vi "KI6221.vi"() -> ()   [LabVIEW 2025] (continued)
                                tunnel: w2439 -> [w2628]
                                tunnel: w2438 -> [w2627]
                                tunnel: w2437 -> [w2626]
                                tunnel: w2436 -> [w2614]
                                tunnel: w2435 -> [w2622]
                                tunnel: [w2620] -> w2433
                                tunnel: w2432 -> [w2619]
                                tunnel: w2430 -> [w2618]
                                tunnel: [w2617] -> w2429
                                tunnel: w2428 -> [w2616]
                                tunnel: w2427 -> [w2615]
                                tunnel: [w2608] -> w2425
                                tunnel: w2421 -> [w2607]
                                tunnel: [w2607] -> w2420
                                tunnel: w2419 -> [w2606]
                                tunnel: [w2605] -> w2410
                                tunnel: [w2604] -> w2418
                                tunnel: [w2603] -> w2417
                                tunnel: [w2598] -> w2416
                                tunnel: w2415 -> [w2598]
                                tunnel: w2406 -> [w2597]
                                frame #0 {
                                # "set STEP source"
                                n1197 = Increment(x=w2465) -> (x+1=w2466:i32)
                                n1198 = case shown="0, Default" w2472 {
                                tunnel: w2471 -> [w2477 _]
                                tunnel: w2470 -> [w2476 _]
                                tunnel: w2469 -> [w2480 w2503]
                                tunnel: w2468 -> [w2479 _]
                                tunnel: [w2478 w2503] -> w2467
                                tunnel: w2464 -> [w2475 _]
                                tunnel: w2466 -> [w2474 _]
                                frame 0, Default {
                                n1199 = case shown="True" w2475 {
                                tunnel: w2480 -> [w2488 w2493]
                                tunnel: w2479 -> [w2487 w2495]
                                tunnel: [w2486 w2494] -> w2478
                                tunnel: w2477 -> [w2484 _]
                                tunnel: w2476 -> [w2483 _]
                                tunnel: w2474 -> [_ w2496]
                                frame False {
                                # "Set Source"
                                n1200 = Number To Exponential String(number=w2488) -> (E-format string=w2491:string)  [unwired: 3 in]
                                n1201 = Initialize Array(w2491, 1 ("dimension size")) -> (w2489:string[])
                                n1202 = call "VisaVarReplace.vi"("Replace Array"=w2489, "Search Array"=string[] ["<LEVEL>"], "GPIB Array"=w2484) -> ("GPIB Array OUT"=w2482:string[])
                                n1203 = call "VISAreadWrite.vi"("GPIB INDEX Array"=i32[] [2], "GPIB ARRAY"=w2482, "VISA REFERENCE"=w2483) -> ("error out 15"=→"error out 23":errorcluster)  [unwired: 1 in, 1 out]
                                n1204 = Add(x=w2488, y=w2487) -> (x+y=w2486:dbl)
                                }
                                frame True {
                                n1205 = Number To Decimal String(number=w2496) -> (decimal integer string=w2498:string)  [unwired: 1 in]
                                n1206 = Number To Engineering String(4:w2493) -> (0:w2497:string)  [unwired: 3 in]
                                n1207 = Concatenate Strings("Please set the external step source for sweep number " ("y"), w2498, ". The correct source setting should be " ("y"), w2497, "." ("string")) -> (w2499:string)
                                n1208 = call "STEP SETUP"("Message"=w2499) -> ()  [unwired: 9 in, 2 out]
                                n1209 = Add(x=w2493, y=w2495) -> (x+y=w2494:dbl)
                                }
                                }
                                }
                                frame 2 {
                                # "No source"
                                }
                                }
                                }
                                frame #1 {
                                # "WORK AUTO TEST or \nFORWARD current values"
                                n1210 = case shown="0, Default" w2522 {
                                tunnel: w2521 -> [w2537 _]
                                tunnel: w2520 -> [_ w2595]
                                tunnel: w2519 -> [_ w2596]
                                tunnel: w2518 -> [_ w2591]
                                tunnel: w2517 -> [w2536 _]
                                tunnel: w2516 -> [w2535 _]
                                tunnel: w2515 -> [w2534 _]
                                tunnel: [w2533 w2592] -> w2514
                                tunnel: [w2532 w2595] -> w2507
                                tunnel: [w2531 w2596] -> w2506
                                tunnel: [w2530 w2591] -> w2513
                                tunnel: w2512 -> [w2529 _]
                                tunnel: w2511 -> [w2528 _]
                                tunnel: w2510 -> [w2527 w2590]
                                tunnel: [w2526 w2590] -> w2509
                                tunnel: [w2525 TRUE ("CONTINUE")] -> w2508
                                tunnel: w2505 -> [w2524 _]
                                tunnel: w2504 -> [w2523 _]
                                frame 0, Default {
                                # "voltage"
                                n1211 = case shown="0, Default" w2537 {
                                tunnel: w2536 -> [w2559 w2588]
                                tunnel: w2535 -> [w2558 w2586]
                                tunnel: w2534 -> [w2557 w2580]
                                tunnel: [w2555 w2581] -> w2533
                                tunnel: [w2549 w2583] -> w2532
                                tunnel: [w2556 w2582] -> w2531
                                tunnel: [w2557 w2580] -> w2530
                                tunnel: w2529 -> [w2554 _]
                                tunnel: w2528 -> [w2553 _]
                                tunnel: w2527 -> [w2552 w2579]
                                tunnel: [w2548 w2579] -> w2526
                                tunnel: [w2547 TRUE ("CONTINUE")] -> w2525
                                tunnel: w2524 -> [w2546 _]
                                tunnel: w2523 -> [w2545 _]
                                frame 0, Default {
                                # "auto test"
                                n1212 = flat-sequence {
                                tunnel: w2553 -> [w2561]
                                tunnel: w2554 -> [w2562]
                                tunnel: w2557 -> [w2563]
                                tunnel: w2558 -> [w2564]
                                tunnel: [w2564] -> w2544
                                tunnel: [w2563] -> w2543
                                tunnel: [w2562] -> w2542
                                tunnel: [w2561] -> w2541
                                tunnel: w2559 -> [w2577]
                                tunnel: [w2574] -> w2556
                                tunnel: [w2573] -> w2555
                                tunnel: [w2572] -> w2539
                                tunnel: w2552 -> [w2569]
                                tunnel: [w2568] -> w2549
                                tunnel: [w2567] -> w2547
                                tunnel: w2546 -> [w2566]
                                tunnel: w2545 -> [w2565]
                                tunnel: w2544 -> [w2576]
                                tunnel: w2543 -> [w2575]
                                tunnel: w2542 -> [w2571]
                                tunnel: w2541 -> [w2570]
                                frame #0 {
                                n1213 = property on="auto test \nlabel" class="Str"("Visible"=TRUE) -> ()  [unwired: 2 in, 2 out]
                                }
                                frame #1 {
                                n1214 = call "autotest.vi"("6220 VISA"=w2571, "start v"=w2577, "stop v"=w2576, "numPTS"=w2575, "GPIB Array"=w2570, "AUTO ARRAY"=w2569, "INIT start I"=w2566, "INIT stop I"=w2565) -> ("start I"=w2568:dbl, "stop I"=w2574:dbl, "step I"=w2573:dbl, "CONTINUE"=w2567:bool, "error out 15"=w2572:errorcluster)  [unwired: 3 in]
                                }
                                }
                                n1215 = property on="auto test label" class="Str"(error in=w2539, "Visible"=FALSE) -> (error out=→"error out 29":errorcluster)  [unwired: 1 in, 1 out]
                                n1216 = Number To Engineering String(4:w2549) -> (0:w2550:string)  [unwired: 3 in]
                                n1217 = Replace Array Subset(array=w2552, new element=w2550, index=4) -> (w2548:string[])
                                }
                                frame 1 {
                                # "estimated res"
                                n1218 = property on="Resistance in Ohms" class="DigNum (strict)"() -> ("Value"=w2587:dbl)  [unwired: 2 in, 2 out]
                                n1219 = Decrement(x=w2580) -> (x-1=w2584:i32)
                                n1220 = Divide(x=w2588, y=w2587) -> (x/y=w2583:dbl)
                                n1221 = Divide(x=w2586, y=w2587) -> (x/y=w2582:dbl)
                                n1222 = Subtract(x=w2582, y=w2583) -> (x-y=w2585:dbl)
                                n1223 = Divide(x=w2585, y=w2584) -> (x/y=w2581:dbl)
                                }
                                }
                                }
                                frame 1 {
                                # "current setup"
                                n1224 = Decrement(x=w2591) -> (x-1=w2593:i32)
                                n1225 = Subtract(x=w2596, y=w2595) -> (x-y=w2594:dbl)
                                n1226 = Divide(x=w2594, y=w2593) -> (x/y=w2592:dbl)
                                }
                                }
                                }
                                frame #2 {
                                # "PING every 3 sec. for all data in buffer. When it is ready grab data, parse into data sheet, and select columns for GRAPHS"
                                # "SEND SCPI CONFIG"
                                # "CREATE VISA SCPI STRINGS"
                                # "DC delta\nsetting\n\nstepsize"
                                # "run sweep"
                                n1227 = Number To Exponential String(number=w2599) -> (E-format string=w2621:string)  [unwired: 3 in]
                                n1228 = Number To Exponential String(number=w2599) -> (E-format string=w2633:string)  [unwired: 3 in]
                                n1229 = local read "Setup String"() -> (w2602:string)
                                n1230 = call "DCONSweepFix.vi"("NUM PTS"=w2614, "STEP"=w2599, "STOP"=w2610, "START"=w2613) -> ("Source Array"=w2609:dbl[], "STOP 2"=w2611:dbl, "START 2"=w2612:dbl)
                                n1231 = Not(x=w2606) -> (.not. x?=w2605:bool)
                                n1232 = Number To Exponential String(number=w2611) -> (E-format string=w2634:string)  [unwired: 3 in]
                                n1233 = Number To Exponential String(number=w2612) -> (E-format string=w2635:string)  [unwired: 3 in]
                                n1234 = Insert Into Array(array=string[] [], new element=w2635) -> (w2645:string[])  [unwired: 1 in]
                                n1235 = Insert Into Array(array=w2645, new element=w2634) -> (w2644:string[])  [unwired: 1 in]
                                n1236 = Insert Into Array(array=w2644, new element=w2633) -> (w2643:string[])  [unwired: 1 in]
                                n1237 = Insert Into Array(array=w2643, new element=w2632) -> (w2639:string[])  [unwired: 1 in]
                                n1238 = Insert Into Array(array=w2639, new element=w2621) -> (w2642:string[])  [unwired: 1 in]
                                n1239 = Insert Into Array(array=w2642, new element=w2631) -> (w2641:string[])  [unwired: 1 in]
                                n1240 = Insert Into Array(array=w2641, new element=w2630) -> (w2640:string[])  [unwired: 1 in]
                                n1241 = Insert Into Array(array=w2640, new element=w2629) -> (w2636:string[])  [unwired: 1 in]
                                n1242 = Insert Into Array(array=w2636, new element=w2628) -> (w2638:string[])  [unwired: 1 in]
                                n1243 = Insert Into Array(array=w2638, new element=w2627) -> (w2637:string[])  [unwired: 1 in]
                                n1244 = Insert Into Array(array=w2637, new element=w2626) -> (w2600:string[])  [unwired: 1 in]
                                n1245 = Insert Into Array(array=w2600, new element=w2602) -> (w2601:string[])  [unwired: 1 in]
                                n1246 = call "VisaVarReplace.vi"("Replace Array"=w2601, "Search Array"=string[] ["<DCONSTART>", "<DCONSTOP>", "<DCONSTEP>", "<DCONDELAY>", "<DCONDELTA>", "<DCONCOMP>", "<DCONDAMPING>", "<DCONVOLTRANGE>", "<DCONNPLC>", "<DCONFILTERSTATE>", "<DCONFILTERCOUNT>", "<SETUPSTRING>"], "GPIB Array"=w2623) -> ("GPIB Array OUT"=w2603:string[])
                                n1247 = case shown="True" w2606 {
                                tunnel: i32[] [24] -> [_ w2653]
                                tunnel: w2603 -> [_ w2652]
                                tunnel: [errorcluster {"status"=FALSE, "code"=0, "source"=""} ("error out 15") w2651] -> w2625
                                tunnel: w2604 -> [_ w2650]
                                frame False {
                                }
                                frame True {
                                n1248 = call "VISAreadWrite.vi"("GPIB INDEX Array"=w2653, "GPIB ARRAY"=w2652, "VISA REFERENCE"=w2650) -> ("error out 15"=w2651:errorcluster)  [unwired: 1 in, 1 out]
                                }
                                }
                                n1249 = case shown="No Error" w2625 {
                                tunnel: [w2672 TRUE ("ABORT DIFF COND")] -> w2624
                                tunnel: w2604 -> [w2671 _]
                                tunnel: w2623 -> [w2670 _]
                                tunnel: w2614 -> [w2669 _]
                                tunnel: w2622 -> [w2668 _]
                                tunnel: w2599 -> [w2667 _]
                                tunnel: [w2666 w2849] -> w2620
                                tunnel: w2619 -> [w2665 w2849]
                                tunnel: w2618 -> [w2664 _]
                                tunnel: [w2663 w2848] -> w2617
                                tunnel: w2616 -> [w2662 w2848]
                                tunnel: w2615 -> [w2661 _]
                                tunnel: w2609 -> [w2660 _]
                                tunnel: [w2659 errorcluster {"status"=FALSE, "code"=0, "source"=""} ("error out")] -> w2608
                                tunnel: w2605 -> [w2658 _]
                                tunnel: w2597 -> [w2656 _]
                                frame No Error {
                                n1250 = Multiply(x=w2656, y=1000.0) -> (x*y=w2655:dbl)
                                n1251 = Wait (ms)(milliseconds to wait=w2655) -> (millisecond timer value=w2654:u32)
                                n1252 = while {
                                tunnel: ["ABORT DIFF COND"] -> w2672
                                tunnel: w2671 -> [w2689]
                                tunnel: w2670 -> [w2688]
                                tunnel: w2669 -> [w2687]
                                tunnel: w2668 -> [w2685]
                                tunnel: w2667 -> [w2684]
                                tunnel: [w2683] -> w2666
                                tunnel: w2665 -> [w2682]
                                tunnel: w2664 -> [w2681]
                                tunnel: [w2680] -> w2663
                                tunnel: w2662 -> [w2679]
                                tunnel: w2661 -> [w2678]
                                tunnel: w2660 -> [w2677]
                                tunnel: [w2676] -> w2659
                                tunnel: w2658 -> [w2673]
                                tunnel: w2654 -> [_]
                                stop <- w2690 stop-if-true
                                n1253 = Or(x=w2673, y="ABORT DIFF COND") -> (x .or. y?=w2674:bool)
                                n1254 = case shown="False" w2674 {
                                selector: w2674 -> [_ w2846]
                                tunnel: w2689 -> [w2707 _]
                                tunnel: w2688 -> [w2706 _]
                                tunnel: w2687 -> [w2705 _]
                                tunnel: [w2702 w2846] -> w2686
                                tunnel: w2685 -> [w2700 _]
                                tunnel: w2684 -> [w2699 _]
                                tunnel: [w2698 w2845] -> w2683
                                tunnel: w2682 -> [w2697 w2845]
                                tunnel: w2681 -> [w2696 _]
                                tunnel: [w2695 w2844] -> w2680
                                tunnel: w2679 -> [w2694 w2844]
                                tunnel: w2678 -> [w2693 _]
                                tunnel: w2677 -> [w2692 _]
                                tunnel: [w2691 errorcluster {"status"=FALSE, "code"=0, "source"=""} ("error out")] -> w2676
                                frame False {
                                n1255 = case shown="True" w2704 {
                                tunnel: w2703 -> [w2716 _]
                                tunnel: [w2715 TRUE] -> w2702
                                tunnel: w2701 -> [_ w2766]
                                tunnel: w2700 -> [_ w2763]
                                tunnel: w2699 -> [_ w2762]
                                tunnel: [w2714 w2749] -> w2698
                                tunnel: w2697 -> [w2714 w2761]
                                tunnel: w2696 -> [_ w2737]
                                tunnel: [w2713 w2734] -> w2695
                                tunnel: w2694 -> [w2713 w2731]
                                tunnel: w2693 -> [_ w2729]
                                tunnel: w2692 -> [_ w2728]
                                tunnel: [w2712 w2724] -> w2691
                                tunnel: [w2711 w2720] -> _
                                tunnel: [w2711 w2719] -> _
                                tunnel: [w2711 w2718] -> _
                                frame False {
                                w2711 = dbl[] []
                                # "NO DATA"
                                n1256 = call "DATA QUERY ERROR"("Enable"=w2716) -> ("error out"=w2712:errorcluster, "Abort test now"=w2715:bool)  [unwired: 9 in]
                                }
                                frame True {
                                # "data"
                                n1257 = property on="Trace offset (% Pk-Pk):" class="DigNum (strict)"() -> ("Value"=w2742:dbl)  [unwired: 2 in, 2 out]
                                n1258 = Multiply(x=6, y=w2737) -> (x*y=w2759:i32)
                                n1259 = Divide(x=w2742, y=100.0) -> (x/y=w2740:dbl)
                                n1260 = Spreadsheet String To Array(delimiter (Tab)=",", format string="%e", spreadsheet string=w2766, array type (2D Dbl)=dbl[] []) -> (array=w2764:dbl[])
                                n1261 = property on="Horizontal Axis:" class="Ring (strict)"() -> ("Value"=w2754:u16)  [unwired: 2 in, 2 out]
                                n1262 = property on="Vertical Axis:" class="Ring (strict)"() -> ("Value"=w2756:u16)  [unwired: 2 in, 2 out]
                                n1263 = Add(x=w2756, y=u16 2) -> (x+y=w2748:u16)
                                n1264 = property on="Differential Conductance Graph" class="XYGraph (strict)"() -> ("Value"=w2757:cluster{"Y":dbl[], "Y":dbl[]}[])  [unwired: 2 in, 2 out]
                                n1265 = Unbundle(w2731) -> (w2733:dbl[], w2732:dbl[], w2730:dbl[])
                                n1266 = while {
                                tunnel: w2764 -> [w2783]
                                shift-right: [w2789] -> w2717
                                shift-left: string[][] [] -> [w2784]
                                tunnel: w2763 -> [w2779]
                                tunnel: w2762 -> [w2777]
                                tunnel: w2728 -> [w2771]
                                i -> [w2773]
                                stop <- w2801 stop-if-true
                                w2780 = "," ("delimiter (Tab)")
                                n1267 = Array Size(array=w2784) -> (size(s)=w2787:i32[])
                                n1268 = Index Array(array=w2787, index=0) -> (element=w2785:i32)
                                n1269 = Multiply(x=5, y=w2785) -> (x*y=w2804:i32)
                                n1270 = Index Array(array=w2783, index=w2804) -> (element=w2778:dbl)
                                n1271 = Divide(x=w2778, y=w2777) -> (x/y=w2776:dbl)
                                n1272 = Increment(x=w2804) -> (x+1=w2802:i32)
                                n1273 = Index Array(array=w2783, index=w2802) -> ()  [unwired: 1 out]
                                n1274 = Increment(x=w2802) -> (x+1=w2803:i32)
                                n1275 = Reciprocal(x=w2776) -> (1/x=w2790:dbl)
                                n1276 = Index Array(array=w2783, index=w2803) -> ()  [unwired: 1 out]
                                n1277 = Index Array(array=w2771, index=w2773) -> (element=w2772:dbl)
                                n1278 = Increment(x=w2803) -> (x+1=w2800:i32)
                                n1279 = Array Size(array=w2783) -> (size(s)=w2788:i32)
                                n1280 = Index Array(array=w2783, index=w2800) -> (element=w2774:dbl)
                                n1281 = Increment(x=w2800) -> (x+1=w2782:i32)
                                n1282 = Number To Engineering String(4:w2772) -> (0:w2794:string)  [unwired: 3 in]
                                n1283 = Number To Engineering String(4:w2776) -> (0:w2792:string)  [unwired: 3 in]
                                n1284 = Number To Engineering String(4:w2790) -> (0:w2791:string)  [unwired: 3 in]
                                n1285 = Number To Engineering String(4:w2778) -> (0:w2793:string)  [unwired: 3 in]
                                n1286 = Number To Engineering String(4:w2779) -> (0:w2775:string)  [unwired: 3 in]
                                n1287 = Number To Engineering String(4:w2774) -> (0:w2795:string)  [unwired: 3 in]
                                n1288 = Index Array(array=w2783, index=w2782) -> ()  [unwired: 1 out]
                                n1289 = Increment(x=w2782) -> (x+1=w2781:i32)
                                n1290 = Concatenate Strings(w2795, w2780, w2794, w2780, w2793, w2780, w2792, w2780, w2791, w2780, w2775) -> (w2796:string)
                                n1291 = Greater Or Equal?(x=w2781, y=w2788) -> (x >= y?=w2801:bool)
                                n1292 = Spreadsheet String To Array(delimiter (Tab)=w2780, format string="%s", spreadsheet string=w2796, array type (2D Dbl)=string[] []) -> (array=w2797:string[])
                                n1293 = Insert Into Array(array=w2784, index (row)=w2773, new element=w2797) -> (w2789:string[][])  [unwired: 1 in]
                                }
                                n1294 = Insert Into Array(array=w2761, index (col)=w2759, new element=w2717) -> (w2749:string[][])  [unwired: 1 in]
                                n1295 = Index Array(array=w2749, index (col)=w2748) -> (element=w2747:string[])  [unwired: 1 in]
                                n1296 = Fract/Exp String To Number(string=w2747) -> (number=w2746:dbl[])  [unwired: 3 in, 1 out]
                                n1297 = Array Max & Min(array=w2746) -> (max value=w2745:dbl, min value=w2744:dbl)  [unwired: 2 out]
                                n1298 = Subtract(x=w2745, y=w2744) -> (x-y=w2743:dbl)
                                n1299 = property on="Differential Conductance Measurement Data" class="Tbl (strict)"("Value"=w2749) -> ()  [unwired: 2 in, 2 out]
                                n1300 = Index Array(array=w2717, index (col)=w2754) -> (element=w2753:string[])  [unwired: 1 in]
                                n1301 = Index Array(array=w2717, index (col)=5 ("disabled index (col)")) -> (element=w2735:string[])  [unwired: 1 in]
                                n1302 = Fract/Exp String To Number(string=w2735) -> (number=w2726:dbl[])  [unwired: 3 in, 1 out]
                                n1303 = Index Array(array=w2717, index (col)=w2748) -> (element=w2752:string[])  [unwired: 1 in]
                                n1304 = Fract/Exp String To Number(string=w2752) -> (number=w2725:dbl[])  [unwired: 3 in, 1 out]
                                n1305 = Multiply(x=w2743, y=w2740) -> (x*y=w2739:dbl)
                                n1306 = Fract/Exp String To Number(string=w2753) -> (number=w2727:dbl[])  [unwired: 3 in, 1 out]
                                n1307 = Insert Into Array(array=w2733, new element=w2727) -> (w2719:dbl[])  [unwired: 1 in]
                                n1308 = Insert Into Array(array=w2732, new element=w2725) -> (w2718:dbl[])  [unwired: 1 in]
                                n1309 = Insert Into Array(array=w2730, new element=w2726) -> (w2720:dbl[])  [unwired: 1 in]
                                n1310 = Multiply(x=w2737, y=w2739) -> (x*y=w2738:dbl)
                                n1311 = Add(x=w2738, y=w2725) -> (x+y=w2750:dbl[])
                                n1312 = To Variant(anything=w2719) -> (Variant=w2722:variant)
                                n1313 = To Variant(anything=w2718) -> (Variant=w2721:variant)
                                n1314 = Bundle(w2727, w2750) -> (w2751:cluster{dbl[], dbl[]})  [unwired: 1 in]
                                n1315 = Insert Into Array(array=w2757, new element=w2751) -> (w2758:cluster{"Y":dbl[], "Y":dbl[]}[])  [unwired: 1 in]
                                n1316 = property on="Differential Conductance Graph" class="XYGraph (strict)"("Value"=w2758) -> ()  [unwired: 2 in, 2 out]
                                n1317 = To Variant(anything=w2720) -> (Variant=w2723:variant)
                                n1318 = Bundle(w2719, w2718, w2720) -> (w2734:cluster{dbl[], dbl[], dbl[]})  [unwired: 1 in]
                                n1319 = call "Stub 3d Graph-4.vi"("Variant"=w2721, "Variant 2"=w2722, "Variant 3"=w2723, "Differential Conductance Surface Plot"=w2729) -> ("error out"=w2724:errorcluster)
                                }
                                }
                                n1320 = flat-sequence {
                                tunnel: w2706 -> [w2808]
                                tunnel: w2707 -> [w2809]
                                tunnel: [w2809] -> w2710
                                tunnel: [w2808] -> w2709
                                tunnel: [w2807] -> w2708
                                tunnel: w2705 -> [w2807]
                                tunnel: [w2822] -> w2701
                                tunnel: w2710 -> [w2821]
                                tunnel: w2709 -> [w2812]
                                tunnel: w2708 -> [w2811]
                                tunnel: [w2814] -> w2704
                                tunnel: [w2813] -> w2703
                                frame #0 {
                                n1321 = Wait (ms)(milliseconds to wait=u32 3000) -> ()  [unwired: 1 out]
                                }
                                frame #1 {
                                n1322 = call "VISAreadWrite.vi"("GPIB INDEX Array"=i32[] [4], "GPIB ARRAY"=w2812, "VISA REFERENCE"=w2821) -> ("error out 15"=w2819:errorcluster, "Read Buffer Array"=w2817:string[])  [unwired: 1 in]
                                n1323 = Index Array(array=w2817, index=1) -> (element=w2816:string)
                                n1324 = Number To Decimal String(number=w2811) -> (decimal integer string=w2810:string)  [unwired: 1 in]
                                n1325 = Decimal String To Number(string=w2816) -> (number=w2815:i32)  [unwired: 2 in, 1 out]
                                n1326 = Less Or Equal?(x=w2811, y=w2815) -> (x <= y?=w2813:bool)
                                n1327 = case shown="True" w2813 {
                                tunnel: ["" w2837] -> w2822
                                tunnel: [FALSE w2836] -> w2814
                                tunnel: w2821 -> [_ w2832]
                                tunnel: w2819 -> [_ w2831]
                                tunnel: w2812 -> [_ w2830]
                                tunnel: w2810 -> [_ w2825]
                                frame False {
                                }
                                frame True {
                                n1328 = Insert Into Array(array=string[] [] ("Replace Array"), new element=w2825) -> (w2826:string[])  [unwired: 1 in]
                                n1329 = call "VisaVarReplace.vi"("Replace Array"=w2826, "Search Array"=string[] ["<DATACOUNT>"], "GPIB Array"=w2830) -> ("GPIB Array OUT"=w2829:string[])
                                n1330 = call "VISAreadWrite.vi"("error in (no error)"=w2831, "GPIB INDEX Array"=i32[] [23], "GPIB ARRAY"=w2829, "VISA REFERENCE"=w2832) -> ("error out 15"=w2834:errorcluster, "Read Buffer Array"=w2835:string[])
                                "error out 25" <- w2834
                                n1331 = Index Array(array=w2835, index=1) -> (element=w2837:string)
                                n1332 = Unbundle(w2834) -> ("source"=w2833:string)  [unwired: 2 out]
                                n1333 = Match Pattern(string=w2833, regular expression="-1073807339") -> (offset past match=w2841:i32)  [unwired: 1 in, 3 out]
                                n1334 = Equal?(x=w2841, y=-1) -> (x = y?=w2836:bool)
                                }
                                }
                                }
                                }
                                }
                                frame True {
                                }
                                }
                                n1335 = Compound Arithmetic op=OR(w2686, "ABORT DIFF COND") -> (w2690:bool)
                                }
                                }
                                frame Error {
                                }
                                }
                                }
                                }
                                n1336 = Decrement(x=w2463) -> (x-1=w2431:i32)
                                n1337 = Greater Or Equal?(x=w2430, y=w2431) -> (x >= y?=w2462:bool)
                                n1338 = Compound Arithmetic op=OR(w2412, w2462, w2410) -> (w2451:bool)
                                n1339 = Or(x=w2410, y=w2412) -> (x .or. y?=w2411:bool)
                                n1340 = Absolute Value(x=w2416) -> (abs(x)=w2408:dbl)
                                n1341 = Absolute Value(x=w2414) -> (abs(x)=w2407:dbl)
                                }
                                n1342 = property on="Main Tabs" class="TabCtl (strict)"(error in=w2236, "Page Selector Visible"=w2235) -> (error out=w2237:errorcluster)  [unwired: 1 in, 1 out]
                                n1343 = property on="Advanced Operation Tab" class="TabCtl (strict)"(error in=w2237, "Page Selector Visible"=w2235) -> (error out=w2279:errorcluster)  [unwired: 1 in, 1 out]
                                n1344 = while {
                                shift-right: [w2367] -> w2299
                                shift-left: string[] [] -> [w2368]
                                tunnel: string[] ["Voltage", "Current", "Delta Voltage", "Resistance", "Conductance", "Step Level"] -> [w2366]
                                tunnel: w2285 -> [w2362]
                                i -> [w2365]
                                stop <- w2363 stop-if-true
                                n1345 = Build Array (concatenate)(w2368, w2366) -> (w2367:string[])
                                n1346 = Increment(x=w2365) -> (x+1=w2364:i32)
                                n1347 = Equal?(x=w2364, y=w2362) -> (x = y?=w2363:bool)
                                }
                                n1348 = case shown="False" w2271 {
                                tunnel: w2279 -> [w2348 w2352]
                                tunnel: [w2348 w2351] -> w2257
                                tunnel: w2278 -> [_ w2350]
                                tunnel: w2277 -> [_ w2349]
                                frame False {
                                }
                                frame True {
                                n1349 = call "VISAreadWrite.vi"("error in (no error)"=w2352, "GPIB INDEX Array"=i32[] [3], "GPIB ARRAY"=w2349, "VISA REFERENCE"=w2350) -> ("error out 15"=w2351:errorcluster)  [unwired: 1 out]
                                }
                                }
                                n1350 = property on="Differential Conductance Measurement Data" class="Tbl (strict)"("Column Header Strings[]"=w2299) -> ()  [unwired: 2 in, 2 out]
                                n1351 = Equal To 0?(x=w2273) -> (x = 0?=w2288:bool)
                                n1352 = Greater?(x=w2285, y=1) -> (0:w2286:bool)
                                n1353 = And(x=w2288, y=w2286) -> (x .and. y?=w2289:bool)
                                n1354 = property on="DC TABS" class="TabCtl (strict)"() -> (error out=w2292:errorcluster, "Pages"=w2295:refnum<vi>[], "Value"=w2282:enum32{"2-D GRAPH", "3-D PLOT", "SHEET", "HELP"})  [unwired: 2 in, 1 out]
                                n1355 = Equal?(x=w2282, y=enum32{"2-D GRAPH", "3-D PLOT", "SHEET", "HELP"}."3-D PLOT") -> (x = y?=w2280:bool)
                                n1356 = case shown="False" w2289 {
                                tunnel: [2 ("y") 0 ("y")] -> w2287
                                tunnel: w2282 -> [w2355 w2360]
                                tunnel: [w2354 w2360] -> w2283
                                tunnel: w2280 -> [w2356 _]
                                frame False {
                                n1357 = case shown="True" w2356 {
                                tunnel: w2355 -> [w2358 _]
                                tunnel: [w2358 0 ("y")] -> w2354
                                frame False {
                                }
                                frame True {
                                }
                                }
                                }
                                frame True {
                                }
                                }
                                n1358 = call "VISAreadWrite.vi"("error in (no error)"=w2257, "GPIB INDEX Array"=i32[] [25], "GPIB ARRAY"=w2254, "VISA REFERENCE"=w2258) -> ("error out 15"=→"error out 32":errorcluster)  [unwired: 1 out]
                                n1359 = case shown="False" w2234 {
                                tunnel: w2244 -> [w2337 _]
                                frame False {
                                n1360 = Array Subset(array=w2337, index (col)=2 ("index"), length (col)=1 ("length")) -> (w2346:string[][])  [unwired: 2 in]
                                n1361 = Fract/Exp String To Number(string=w2346) -> (number=w2345:dbl[][])  [unwired: 3 in, 1 out]
                                n1362 = Array Max & Min(array=w2345) -> (max value=w2340:dbl, min value=w2344:dbl)  [unwired: 2 out]
                                n1363 = Greater?(x=w2340, y=1e+30) -> (0:w2338:bool)
                                n1364 = call "Volt range problem"("Enable"=w2338) -> ()  [unwired: 9 in, 2 out]
                                n1365 = Equal To 0?(x=w2340) -> (x = 0?=w2342:bool)
                                n1366 = Equal?(x=w2344, y=w2340) -> (x = y?=w2343:bool)
                                n1367 = And(x=w2343, y=w2342) -> (x .and. y?=w2341:bool)
                                n1368 = call "Volt range problem"("Enable"=w2341) -> ()  [unwired: 9 in, 2 out]
                                }
                                frame True {
                                }
                                }
                                n1369 = Index Array(array=w2295, index=1) -> (element=w2293:refnum<vi>)
                                n1370 = property class="Page"(reference=w2293, error in=w2292, "Page Enabled State"=w2287) -> (error out=w2291:errorcluster)  [unwired: 1 out]
                                n1371 = property on="DC TABS" class="TabCtl (strict)"(error in=w2291, "Value"=w2283) -> (error out=→"error out 30":errorcluster)  [unwired: 1 in, 1 out]
                              }
                            }
                          }
                        }
                      }
                      frame True {
                        # "DEMO MODE"
                        n1372 = property on="I want to control my\n test in terms of:" class="Ring (strict)"() -> ("Value"=w2862:u16)  [unwired: 2 in, 2 out]
                        n1373 = property on="Number of steps" class="DigNum (strict)"() -> ("Value"=w2861:i32)  [unwired: 2 in, 2 out]
                        n1374 = case shown="1" w2862 {
                          tunnel: [w2870 w2871] -> w2853
                          frame 0, Default {
                            n1375 = property on="Number of\n sweep points" class="DigNum (strict)"() -> ("Value"=w2870:i32)  [unwired: 2 in, 2 out]
                          }
                          frame 1 {
                            n1376 = property on="Number of\n sweep points" class="DigNum (strict)"() -> ("Value"=w2871:i32)  [unwired: 2 in, 2 out]
                          }
                        }
                        n1377 = Array Size(array=w2860) -> (size(s)=w2859:i32[])
                        n1378 = Index Array(array=w2859, index=0) -> (element=w2856:i32)
                        n1379 = Index Array(array=w2859, index=1) -> (element=w2855:i32)
                        n1380 = Initialize Array("", w2856, w2855) -> (w2863:string[][])
                        n1381 = while {
                          tunnel: w2869 -> [w2892]
                          tunnel: w2868 -> [w2877]
                          tunnel: w2860 -> [w2883]
                          tunnel: w2867 -> [w2891]
                          shift-right: [w2885] -> _
                          shift-left: w2863 -> [w2886]
                          tunnel: w2861 -> [w2873]
                          tunnel: w2854 -> [w2876]
                          tunnel: cluster{"Y":dbl[], "Y":dbl[]}[] [] ("XY Graph") -> [w2888]
                          tunnel: dbl[][] [] -> [w2884]
                          tunnel: w2853 -> [_]
                          tunnel: w2852 -> [w2874]
                          i -> [w2881]
                          stop <- w2889 stop-if-true
                          w2879 = 6 ("y")
                          n1382 = Multiply(x=w2881, y=w2879) -> (x*y=w2880:i32)
                          n1383 = Array Subset(array=w2883, index (col)=w2880, length (col)=w2879) -> (w2882:string[][])  [unwired: 2 in]
                          n1384 = Add(x=u16 2, y=w2892) -> (x+y=w2878:u16)
                          n1385 = Index Array(array=w2882, index (col)=w2877) -> (element=w2895:string[])  [unwired: 1 in]
                          n1386 = Index Array(array=w2882, index (col)=w2878) -> (element=w2894:string[])  [unwired: 1 in]
                          n1387 = Array Size(array=w2894) -> (size(s)=w2893:i32)
                          n1388 = case shown="True" w2891 {
                            tunnel: [u16 0 ("x") w2907] -> w2890
                            tunnel: [w2900 w2902] -> w2875
                            tunnel: string[] ["Voltage", "Current", "Delta Voltage", "Resistance", "Conductance", "Step Level"] -> [w2898 w2905]
                            tunnel: string[] [] -> [_ w2904]
                            tunnel: w2873 -> [w2897 w2903]
                            frame False {
                              n1389 = property on="Differential Conductance Measurement Data" class="Tbl (strict)"("Column Header Strings[]"=w2898) -> ()  [unwired: 2 in, 2 out]
                              n1390 = Initialize Array(0.0 ("x"), w2897) -> (w2900:dbl[])
                            }
                            frame True {
                              n1391 = while {
                                shift-right: [w2917] -> w2906
                                shift-left: w2904 -> [w2918]
                                tunnel: w2905 -> [w2916]
                                tunnel: w2903 -> [w2912]
                                i -> [w2915]
                                stop <- w2913 stop-if-true
                                n1392 = Build Array (concatenate)(w2918, w2916) -> (w2917:string[])
                                n1393 = Increment(x=w2915) -> (x+1=w2914:i32)
                                n1394 = Equal?(x=w2914, y=w2912) -> (x = y?=w2913:bool)
                              }
                              n1395 = property on="Differential Conductance \nMeasurement Data" class="Tbl (strict)"("Column Header Strings[]"=w2906) -> ()  [unwired: 2 in, 2 out]
                              n1396 = property on="Start Level" class="DigNum (strict)"() -> ("Value"=w2909:dbl)  [unwired: 2 in, 2 out]
                              n1397 = property on="Stop Level" class="DigNum (strict)"() -> ("Value"=w2911:dbl)  [unwired: 2 in, 2 out]
                              n1398 = while {
                                tunnel: w2909 -> [w2924]
                                shift-right: [w2931] -> w2902
                                shift-left: dbl[] [] -> [w2930]
                                tunnel: w2911 -> [w2929]
                                tunnel: w2903 -> [w2928]
                                i -> [w2921]
                                stop <- w2922 stop-if-true
                                n1399 = Subtract(x=w2928, y=1) -> (x-y=w2920:i32)
                                n1400 = Subtract(x=w2929, y=w2924) -> (x-y=w2926:dbl)
                                n1401 = Divide(x=w2926, y=w2920) -> (x/y=w2925:dbl)
                                n1402 = Multiply(x=w2925, y=w2921) -> (x*y=w2923:dbl)
                                n1403 = Add(x=w2924, y=w2923) -> (x+y=w2919:dbl)
                                n1404 = Insert Into Array(array=w2930, index=w2921, new element=w2919) -> (w2931:dbl[])
                                n1405 = Equal?(x=w2920, y=w2921) -> (x = y?=w2922:bool)
                              }
                              n1406 = Subtract(x=w2903, y=1) -> (x-y=w2907:i32)
                            }
                          }
                          n1407 = case shown="1, Default" w2893 {
                            tunnel: w2895 -> [_ w2960]
                            tunnel: w2894 -> [_ w2959]
                            tunnel: w2893 -> [_ w2958]
                            tunnel: w2882 -> [_ w2957]
                            tunnel: w2875 -> [_ w2956]
                            tunnel: w2888 -> [_ w2955]
                            tunnel: w2881 -> [_ w2953]
                            tunnel: [w2932 w2939] -> w2885
                            tunnel: w2886 -> [w2932 w2951]
                            tunnel: w2884 -> [_ w2954]
                            tunnel: w2878 -> [_ w2938]
                            tunnel: w2877 -> [_ w2937]
                            tunnel: w2877 -> [_ w2952]
                            tunnel: w2876 -> [_ w2950]
                            tunnel: w2874 -> [_ w2946]
                            tunnel: w2873 -> [_ w2936]
                            frame 0 {
                            }
                            frame 1, Default {
                              w2940 = string[] []
                              w2948 = 5 items=["cwLine"=1, "cwPoint"=2, "cwLinePoint"=3, "cwHiddenLine"=4, "cwSurface"=5, "cwSurfaceLine"=6, "cwSurfaceNormal"=7, "cwContourLine"=8, "cwSurfaceContour"=9] ("plot style")
                              n1408 = while {
                                tunnel: w2960 -> [_] mode=indexing
                                tunnel: w2959 -> [_] mode=indexing
                                tunnel: w2958 -> [w3005]
                                shift-right: [w2983] -> w2939
                                shift-left: w2951 -> [w3001]
                                tunnel: [w3003] -> _
                                tunnel: w2957 -> [w3002]
                                tunnel: w2956 -> [w2984]
                                tunnel: w2953 -> [w2991]
                                tunnel: w2953 -> [_]
                                tunnel: w2938 -> [w2993]
                                tunnel: w2937 -> [_]
                                tunnel: w2952 -> [w2992]
                                tunnel: w2955 -> [w2990]
                                tunnel: w2954 -> [w2988]
                                tunnel: w2950 -> [w2989]
                                tunnel: [w2987] -> w2949
                                tunnel: [w2986] -> _
                                tunnel: [w2985] -> _
                                tunnel: [w2984] -> _
                                i -> [w2994]
                                stop <- w3004 stop-if-true
                                # "zeros\nper inner\nouters\nsaved"
                                # "offset"
                                # "num step"
                                # "Y"
                                # "X"
                                n1409 = Decrement(x=w3005) -> (x-1=w3007:i32)
                                n1410 = Index Array(array=w3002, index (row)=w2994) -> (element=w2997:string[])  [unwired: 1 in]
                                n1411 = Equal?(x=w3007, y=w2994) -> (x = y?=w3000:bool)
                                n1412 = Index Array(array=w3001, index (row)=w2994) -> (element=w2998:string[])  [unwired: 1 in]
                                n1413 = Wait (ms)(milliseconds to wait=u16 10 ("x")) -> ()  [unwired: 1 out]
                                n1414 = Search 1D Array(1D array=w2998, element="") -> (index of element=w2996:i32)  [unwired: 1 in]
                                n1415 = Replace Array Subset(array=w2998, new element=w2997, index=w2996) -> (w2995:string[])
                                n1416 = Replace Array Subset(array=w3001, new element=w2995, index (row)=w2994) -> (w2983:string[][])  [unwired: 1 in]
                                "Differential Conductance Measurement Data" <- w2983
                                n1417 = while {
                                tunnel: w2983 -> [w3026]
                                tunnel: w2993 -> [w3037]
                                tunnel: w2992 -> [w3035]
                                tunnel: w2991 -> [w3019]
                                shift-right: [w3016] -> w2987
                                shift-left: w2990 -> [w3030]
                                tunnel: w2989 -> [w3010]
                                tunnel: [w3018] -> w2986
                                tunnel: w2988 -> [w3017]
                                tunnel: [w3014] -> w2985
                                i -> [w3020]
                                stop <- w3032 stop-if-true
                                n1418 = Multiply(x=6, y=w3020) -> (x*y=w3033:i32)
                                n1419 = Add(x=w3035, y=w3033) -> (x+y=w3034:i32)
                                n1420 = Add(x=w3037, y=w3033) -> (x+y=w3021:i32)
                                n1421 = Index Array(array=w3026, index (col)=w3021) -> (element=w3022:string[])  [unwired: 1 in]
                                n1422 = Search 1D Array(1D array=w3022, element="") -> (index of element=w3024:i32)  [unwired: 1 in]
                                n1423 = case shown="0, Default" w3024 {
                                selector: w3024 -> [w3046 _]
                                tunnel: [w3046 w3048] -> w3023
                                tunnel: w3022 -> [_ w3047]
                                frame 0, Default {
                                }
                                frame -1 {
                                n1424 = Array Size(array=w3047) -> (size(s)=w3048:i32)
                                }
                                }
                                n1425 = Array Subset(array=w3026, length (row)=w3023) -> (w3025:string[][])  [unwired: 3 in]
                                n1426 = Fract/Exp String To Number(string=w3025) -> (number=w3038:dbl[][])  [unwired: 3 in, 1 out]
                                n1427 = Index Array(array=w3038, index (col)=w3021) -> (element=w3008:dbl[])  [unwired: 1 in]
                                n1428 = Array Max & Min(array=w3008) -> (max value=w3012:dbl, min value=w3013:dbl)  [unwired: 2 out]
                                n1429 = Index Array(array=w3038, index (col)=w3034) -> (element=w3014:dbl[])  [unwired: 1 in]
                                n1430 = Subtract(x=w3012, y=w3013) -> (x-y=w3011:dbl)
                                n1431 = Multiply(x=w3011, y=w3010) -> (x*y=w3009:dbl)
                                n1432 = Multiply(x=w3009, y=w3020) -> (x*y=w3028:dbl)
                                n1433 = Equal?(x=w3019, y=w3020) -> (x = y?=w3032:bool)
                                n1434 = Add(x=w3008, y=w3028) -> (x+y=w3029:dbl[])
                                n1435 = Bundle(w3014, w3029) -> (w3031:cluster{dbl[], dbl[]})  [unwired: 1 in]
                                n1436 = Insert Into Array(array=w3030, index=w3020, new element=w3031) -> (w3016:cluster{"Y":dbl[], "Y":dbl[]}[])
                                n1437 = Array Size(array=w3016) -> (size(s)=w3015:i32)
                                n1438 = while {
                                shift-right: [w3045] -> w3018
                                shift-left: w3017 -> [w3044]
                                tunnel: w3015 -> [w3041]
                                tunnel: w3008 -> [w3039]
                                i -> [w3042]
                                stop <- w3043 stop-if-true
                                n1439 = Decrement(x=w3041) -> (x-1=w3040:i32)
                                n1440 = Build Array (concatenate)(w3044, w3039) -> (w3045:dbl[][])
                                n1441 = Equal?(x=w3042, y=w3040) -> (x = y?=w3043:bool)
                                }
                                }
                                n1442 = property on="ABORT DIFF COND" class="Bool (strict)"() -> ("Value"=w3003:bool)  [unwired: 2 in, 2 out]
                                n1443 = Or(x=w3003, y=w3000) -> (x .or. y?=w3004:bool)
                              }
                              n1444 = while {
                                tunnel: w2939 -> [w2980]
                                shift-right: [w2973] -> w2941
                                shift-left: w2940 -> [w2970]
                                shift-right: [w2972] -> w2942
                                shift-left: w2940 -> [w2969]
                                shift-right: [w2971] -> w2943
                                shift-left: w2940 -> [w2968]
                                tunnel: w2938 -> [w2966]
                                tunnel: w2937 -> [w2965]
                                tunnel: w2936 -> [w2962]
                                i -> [w2963]
                                stop <- w2964 stop-if-true
                                n1445 = Multiply(x=6, y=w2963) -> (x*y=w2981:i32)
                                n1446 = Add(x=w2965, y=w2981) -> (x+y=w2979:i32)
                                n1447 = Add(x=w2966, y=w2981) -> (x+y=w2978:i32)
                                n1448 = Add(x=5, y=w2981) -> (x+y=w2977:i32)
                                n1449 = Index Array(array=w2980, index (col)=w2979) -> (element=w2976:string[])  [unwired: 1 in]
                                n1450 = Index Array(array=w2980, index (col)=w2978) -> (element=w2975:string[])  [unwired: 1 in]
                                n1451 = Index Array(array=w2980, index (col)=w2977) -> (element=w2974:string[])  [unwired: 1 in]
                                n1452 = Decrement(x=w2962) -> (x-1=w2961:i32)
                                n1453 = Build Array (concatenate)(w2970, w2976) -> (w2973:string[])
                                n1454 = Build Array (concatenate)(w2969, w2975) -> (w2972:string[])
                                n1455 = Build Array (concatenate)(w2968, w2974) -> (w2971:string[])
                                n1456 = Equal?(x=w2961, y=w2963) -> (x = y?=w2964:bool)
                              }
                              n1457 = property on="Differential \nConductance Graph" class="XYGraph (strict)"("Value"=w2949) -> ()  [unwired: 2 in, 2 out]
                              n1458 = call "Basic Properties.vi"("Differential Conductance Surface Plot"=w2946, "fast draw"=TRUE, "plot style"=w2948) -> ("3D graph out"=w2945:refnum<k7>, "error out"=w2944:errorcluster)  [unwired: 11 in]
                              n1459 = Fract/Exp String To Number(string=w2941) -> (number=w2933:dbl[])  [unwired: 3 in, 1 out]
                              n1460 = Fract/Exp String To Number(string=w2942) -> (number=w2934:dbl[])  [unwired: 3 in, 1 out]
                              n1461 = Fract/Exp String To Number(string=w2943) -> (number=w2935:dbl[])  [unwired: 3 in, 1 out]
                              n1462 = call "Stub 3D Graph-1.vi"("Array"=w2933, "error out"=w2944, "Array 2"=w2934, "Array 3"=w2935, "3D graph out"=w2945) -> ()
                            }
                          }
                          n1463 = Equal?(x=w2890, y=w2881) -> (x = y?=w2889:bool)
                        }
                      }
                    }
                    n1464 = property on="Vertical Axis:" class="Ring (strict)"(error in=w2112, "Disabled"=w2130) -> (error out=w2119:errorcluster)  [unwired: 1 in, 1 out]
                    n1465 = property on="Horizontal Axis:" class="Ring (strict)"(error in=w2119, "Disabled"=w2130) -> (error out=w2120:errorcluster)  [unwired: 1 in, 1 out]
                    n1466 = property on="Trace offset (% Pk-Pk):" class="DigNum (strict)"(error in=w2120, "Disabled"=w2130) -> ()  [unwired: 1 in, 2 out]
                    n1467 = property on="ABORT DIFF COND" class="Bool (strict)"(error in=w2120, "Value"=FALSE ("ABORT DIFF COND"), "Disabled"=2) -> (error out=w2134:errorcluster)  [unwired: 1 in, 1 out]
                    n1468 = property on="RUN DIFF COND" class="Bool"(error in=w2134, "Disabled"=w2130) -> (error out=w2116:errorcluster)  [unwired: 1 in, 1 out]
                    n1469 = property on="Advanced Operation Tab" class="TabCtl (strict)"(error in=w2116, "Page Selector Visible"=w2117) -> (error out=w2115:errorcluster)  [unwired: 1 in, 1 out]
                    n1470 = property on="Main Tabs" class="TabCtl (strict)"(error in=w2115, "Page Selector Visible"=w2117) -> ()  [unwired: 1 in, 2 out]
                  }
                }
                n1471 = case shown="False" w1866 {
                  tunnel: w1886 -> [w2010 _]
                  tunnel: w1885 -> [w2030 _]
                  tunnel: w1884 -> [w2032 _]
                  tunnel: w1883 -> [w2031 _]
                  tunnel: "Differential Conductance Surface Plot" -> [w2015 _]
                  tunnel: w1846 -> [w2004 _]
                  tunnel: w1847 -> [w2002 _]
                  frame False {
                    w2011 = string[] []
                    (unwired) 1.0 ("Trace offset:")
                    w2016 = 5 items=["cwLine"=1, "cwPoint"=2, "cwLinePoint"=3, "cwHiddenLine"=4, "cwSurface"=5, "cwSurfaceLine"=6, "cwSurfaceNormal"=7, "cwContourLine"=8, "cwSurfaceContour"=9] ("plot style")
                    # "HOR AX"
                    # "i out"
                    # "offset"
                    n1472 = property on="OFFSET DC LAST" class="DigNum (strict)"("Value"=w2002) -> ()  [unwired: 2 in, 2 out]
                    n1473 = property on="X AXIS LAST -DC" class="DigNum (strict)"("Value"=w2010) -> ()  [unwired: 2 in, 2 out]
                    n1474 = property on="Y AXIS LAST -DC" class="DigNum (strict)"("Value"=w2030) -> ()  [unwired: 2 in, 2 out]
                    n1475 = Add(x=w2030, y=2) -> (x+y=w2009:i32)
                    n1476 = Array Size(array=w2004) -> (size(s)=w2027:i32[])
                    n1477 = Index Array(array=w2027, index=1) -> (element=w2025:i32)
                    n1478 = Index Array(array=w2031, index=w2030) -> (element=w2018:string)
                    n1479 = Divide(x=w2002, y=100.0) -> (x/y=w2024:dbl)
                    n1480 = Index Array(array=w2032, index=w2010) -> (element=w2019:string)
                    n1481 = property on="Differential Conductance Graph" class="XYGraph (strict)"("X Scale.Name Label.Text"=w2019, "Y Scale.Name Label.Text"=w2018) -> ()  [unwired: 2 in, 2 out]
                    n1482 = while {
                      shift-right: [w2090] -> w2001
                      shift-left: cluster{"Y":dbl[], "Y":dbl[]}[] [] ("XY Graph") -> [w2097]
                      tunnel: [w2091] -> _
                      tunnel: [w2088] -> _
                      tunnel: w2004 -> [w2087]
                      tunnel: dbl[][] [] -> [w2086]
                      tunnel: w2025 -> [w2072]
                      tunnel: w2010 -> [w2085]
                      tunnel: w2009 -> [w2075]
                      tunnel: w2024 -> [w2078]
                      i -> [w2092]
                      stop <- w2099 stop-if-true
                      w2073 = 6 ("x")
                      n1483 = Multiply(x=w2073, y=w2092) -> (x*y=w2069:i32)
                      n1484 = Add(x=w2085, y=w2069) -> (x+y=w2100:i32)
                      n1485 = Add(x=w2069, y=w2075) -> (x+y=w2070:i32)
                      n1486 = Index Array(array=w2087, index (col)=w2070) -> (element=w2093:string[])  [unwired: 1 in]
                      n1487 = Search 1D Array(1D array=w2093, element="") -> (index of element=w2095:i32)  [unwired: 1 in]
                      n1488 = Divide(x=w2072, y=w2073) -> (x/y=w2074:dbl)
                      n1489 = case shown="-1" w2095 {
                        selector: w2095 -> [w2109 _]
                        tunnel: [w2109 w2111] -> w2094
                        tunnel: w2093 -> [_ w2110]
                        frame 0, Default {
                        }
                        frame -1 {
                          n1490 = Array Size(array=w2110) -> (size(s)=w2111:i32)
                        }
                      }
                      n1491 = Array Subset(array=w2087, length (row)=w2094) -> (w2084:string[][])  [unwired: 3 in]
                      n1492 = Fract/Exp String To Number(string=w2084) -> (number=w2101:dbl[][])  [unwired: 3 in, 1 out]
                      n1493 = Index Array(array=w2101, index (col)=w2100) -> (element=w2088:dbl[])  [unwired: 1 in]
                      n1494 = Index Array(array=w2101, index (col)=w2070) -> (element=w2081:dbl[])  [unwired: 1 in]
                      n1495 = Array Max & Min(array=w2081) -> (max value=w2079:dbl, min value=w2080:dbl)  [unwired: 2 out]
                      n1496 = Subtract(x=w2079, y=w2080) -> (x-y=w2077:dbl)
                      n1497 = Multiply(x=w2077, y=w2078) -> (x*y=w2076:dbl)
                      n1498 = Multiply(x=w2076, y=w2092) -> (x*y=w2096:dbl)
                      n1499 = Add(x=w2081, y=w2096) -> (x+y=w2083:dbl[])
                      n1500 = Bundle(w2088, w2083) -> (w2098:cluster{dbl[], dbl[]})  [unwired: 1 in]
                      n1501 = Insert Into Array(array=w2097, index=w2092, new element=w2098) -> (w2090:cluster{"Y":dbl[], "Y":dbl[]}[])
                      n1502 = Array Size(array=w2090) -> (size(s)=w2089:i32)
                      n1503 = Decrement(x=w2074) -> (x-1=w2071:dbl)
                      n1504 = while {
                        shift-right: [w2108] -> w2091
                        shift-left: w2086 -> [w2107]
                        tunnel: w2089 -> [w2104]
                        tunnel: w2081 -> [w2102]
                        i -> [w2105]
                        stop <- w2106 stop-if-true
                        n1505 = Decrement(x=w2104) -> (x-1=w2103:i32)
                        n1506 = Build Array (concatenate)(w2107, w2102) -> (w2108:dbl[][])
                        n1507 = Equal?(x=w2105, y=w2103) -> (x = y?=w2106:bool)
                      }
                      n1508 = Equal?(x=w2071, y=w2092) -> (x = y?=w2099:bool)
                    }
                    "Differential Conductance Graph" <- w2001
                    n1509 = property on="Number of steps" class="DigNum (strict)"() -> ("Value"=w2008:i32)  [unwired: 2 in, 2 out]
                    n1510 = property on="Start Level" class="DigNum (strict)"() -> ("Value"=w2020:dbl)  [unwired: 2 in, 2 out]
